vi "setDevice.vi"(8 "error in (no error)":errorcluster, 10 "Device.lvclass":refnum<class "Device.lvclass">, 11 "BasicRemote in":refnum<class "BasicRemote.lvclass">) -> (0 "error out":errorcluster, 3 "BasicRemote out":refnum<class "BasicRemote.lvclass">)   [LabVIEW 2017, in "BasicRemote.lvclass"]
uses:
  BasicRemote.lvclass
  Device Class/Device.lvclass
  BasicRemote.lvclass/BasicRemote.ctl
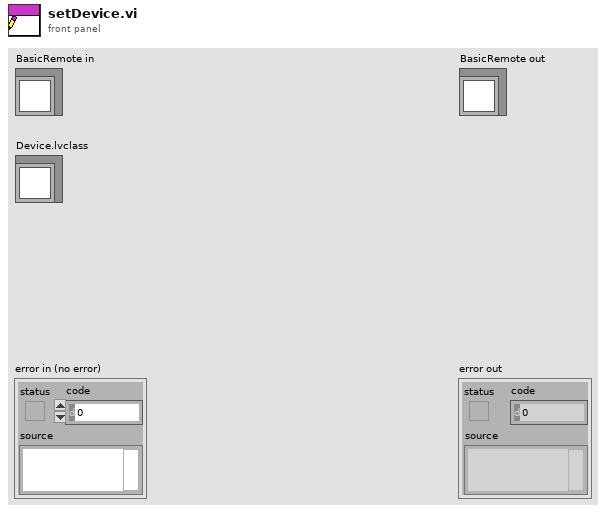
[diagram p1: front panel]
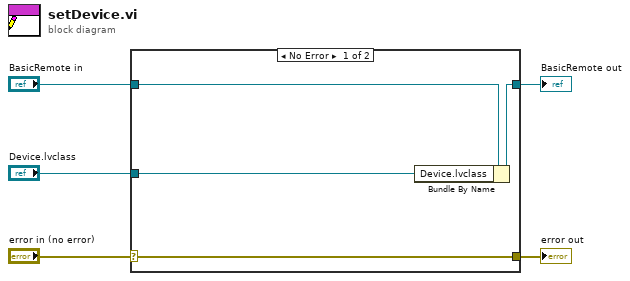
[diagram p0: block diagram]
diagram:
  n1 = case shown="No Error" "error in (no error)" {
    selector: "error in (no error)" -> [w9 w10]
    tunnel: [w9 w10] -> w4
    tunnel: [w7 w11] -> w2
    tunnel: "BasicRemote in" -> [w8 w11]
    tunnel: "Device.lvclass" -> [w6 _]
    frame No Error {
      n2 = Bundle By Name(cluster=w8, "Device.lvclass"=w6) -> (w7:refnum<class "BasicRemote.lvclass">)
    }
    frame Error {
    }
  }
  "error out" <- w4
  "BasicRemote out" <- w2
